vi "removeDeviceFromHWList.vi"(8 "error in (no error)":errorcluster, 10 "deviceName":string, 11 "HWController in":refnum<class "HWController.lvclass">) -> (0 "error out":errorcluster, 3 "HWController out":refnum<class "HWController.lvclass">)   [LabVIEW 2009, in "Hardware.lvlib" / "HWControllers.lvlib" / "HWController.lvclass"]
uses:
  HWController.lvclass
  HWController.lvclass/HWController.ctl
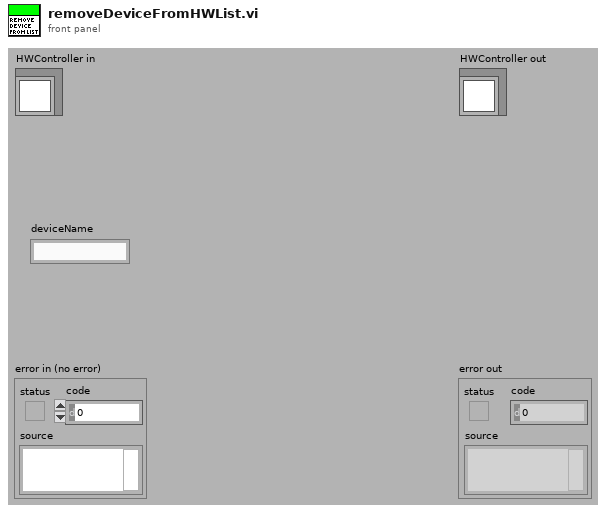
[diagram p1: front panel]
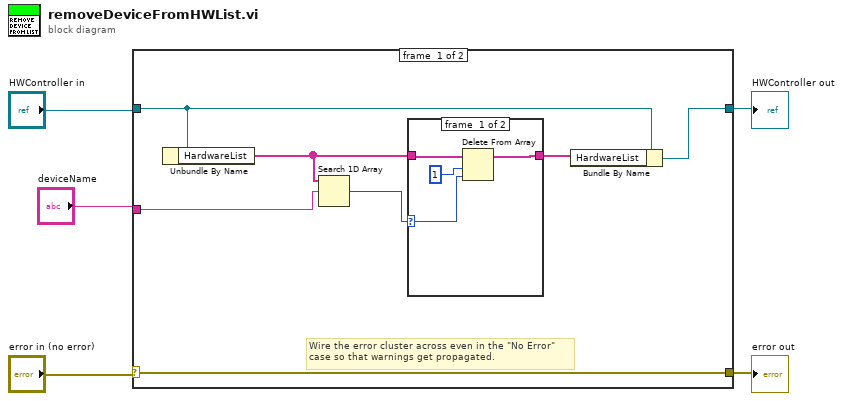
[diagram p0: block diagram]
diagram:
  n1 = case shown="No Error" "error in (no error)" {
    selector: "error in (no error)" -> [w12 w19]
    tunnel: [w12 w19] -> w1
    tunnel: [w10 w18] -> w2
    tunnel: "HWController in" -> [w11 w18]
    tunnel: "deviceName" -> [w9 _]
    frame #0 {
      # "Wire the error cluster across even in the \"No Error\"\ncase so that warnings get propagated."
      n2 = Unbundle By Name(w11) -> ("HardwareList"=w7:string[])
      n3 = Search 1D Array(1D array=w7, element=w9) -> (index of element=w8:i32)  [unwired: 1 in]
      n4 = case shown="-1" w8 {
        selector: w8 -> [w14 _]
        tunnel: w7 -> [w16 w17]
        tunnel: [w15 w17] -> w6
        frame #0 {
          n5 = Delete From Array(array=w16, length=1, index=w14) -> (array with subset deleted=w15:string[])  [unwired: 1 out]
        }
        frame #1 {
        }
      }
      n6 = Bundle By Name(cluster=w11, "HardwareList"=w6) -> (w10:refnum<class "HWController.lvclass">)
    }
    frame #1 {
    }
  }
  "error out" <- w1
  "HWController out" <- w2
